vi "MongoDB.FindandModify.vi"(8 "error in (no error)":errorcluster, 11 "MongoDB.Collection in":refnum<class "MongoDB.Collection.lvclass">) -> (0 "error out":errorcluster, 3 "MongoDB.Collection out":refnum<class "MongoDB.Collection.lvclass">)   [LabVIEW 2014, in "MongoDB.Collection.lvclass"]
uses:
  MongoDB.Collection.lvclass
  C:/Users/Richard/Documents/GitHub/mongo-labview-driver/CSharp/bin/MongoDB.Driver.Legacy.dll
  CSharp/bin/MongoDB.Driver.Legacy.dll
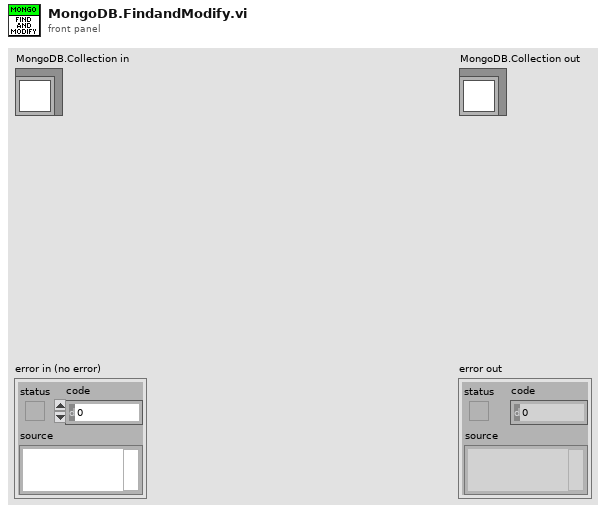
[diagram p1: front panel]
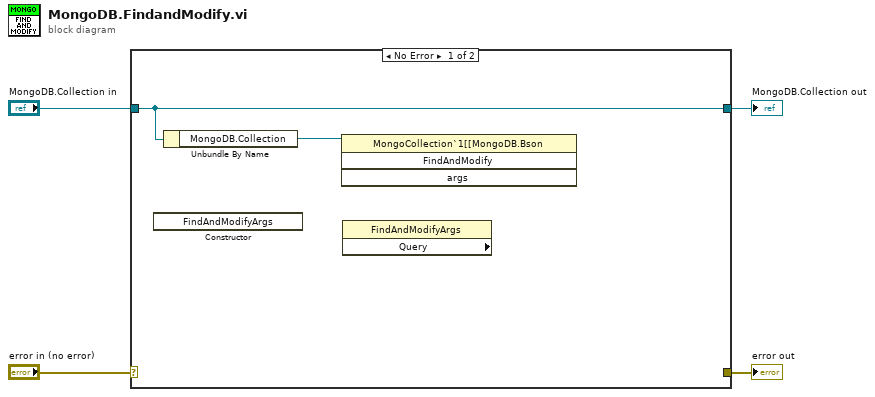
[diagram p0: block diagram]
diagram:
  n1 = case shown="No Error" "error in (no error)" {
    selector: "error in (no error)" -> [_ w8]
    tunnel: [_ w8] -> w3
    tunnel: [w6 w7] -> w1
    tunnel: "MongoDB.Collection in" -> [w6 w7]
    frame No Error {
      n2 = constructor class="FindAndModifyArgs"() -> ()  [unwired: 3 in, 3 out]
      n3 = Unbundle By Name(w6) -> ("MongoDB.Collection"=w5:refnum<k24>)
      n4 = invoke class="MongoCollection`1[[MongoDB.Bson" method="FindAndModify"(reference=w5) -> ()  [unwired: 3 in, 4 out]
      n5 = property class="FindAndModifyArgs" props=["Query"]() -> ()  [unwired: 2 in, 3 out]
    }
    frame Error {
    }
  }
  "error out" <- w3
  "MongoDB.Collection out" <- w1
